vi "RoboticArm_Dashboard.vi"() -> ()   [LabVIEW 2019]
uses:
  <vilib>/MakerHub/Xbox-One-Controller/Public/Open by Index.vi
  <vilib>/vision/driver/NI_Vision_Acquisition_Software.lvlib
  <vilib>/MakerHub/Xbox-One-Controller/Private/Type Defs/Indicators/All Buttons Visual.ctl
  <vilib>/MakerHub/Xbox-One-Controller/Private/Type Defs/Indicators/A.ctl
  <vilib>/MakerHub/Xbox-One-Controller/Private/Type Defs/Indicators/B.ctl
  <vilib>/MakerHub/Xbox-One-Controller/Private/Type Defs/Indicators/X.ctl
  <vilib>/MakerHub/Xbox-One-Controller/Private/Type Defs/Indicators/Y.ctl
  <vilib>/MakerHub/Xbox-One-Controller/Private/Type Defs/Indicators/View.ctl
  <vilib>/MakerHub/Xbox-One-Controller/Private/Type Defs/Indicators/Menu.ctl
  <vilib>/MakerHub/Xbox-One-Controller/Private/Type Defs/Indicators/Thumbstick.ctl
  <vilib>/MakerHub/Xbox-One-Controller/Private/Type Defs/Indicators/Left Bumper.ctl
  <vilib>/MakerHub/Xbox-One-Controller/Private/Type Defs/Indicators/Right Bumper.ctl
  <vilib>/MakerHub/Xbox-One-Controller/Private/Type Defs/Indicators/All Axis Data.ctl
  <vilib>/MakerHub/Xbox-One-Controller/Private/Type Defs/Indicators/DPad Enum.ctl
  <vilib>/userDefined/High Color/IMAQdx.ctl
panel:
  in  "Session In":T1
  in  "Stop 2":bool
  out "Frame Rate":dbl(knob) scale=0.0..100.0
  out "Image":T2(plugin-control)
  out "Buffer Number":u32
  in  "Tab Control":T3(tab)
  in  "Blank Button":bool
  in  "PORT":dbl
  in  "IP-ADDRESS":string(combo)
  in  "Stop":bool
  in  "TCP/IP control":bool
  out "Servos Software Control":u8[](array[numeric])
  out "Manual?":bool
  in  "Servo control":bool
  out "Register values":i32[](array[numeric])
  in  "Servos manual angle":u8[](array[numeric])
  out "Value sent to Raspberry Pi":string
  out "hex integer string":string[](array[string])
  out "Raspberry pi feedback":string
  out "Stop?":bool
  out "Socket Error Out":errorcluster
  out "Gamepad Error Out":errorcluster
  out "Buttons":T4
  out "All Axis":T14
  in  "Device Index":i32
  in  "link B":dbl
  in  "link A":dbl
  out "Servo A":dbl(knob) scale=0.0..180.0
  in  "dist":dbl(knob) scale=50.0..250.0
  out "Servo B":dbl(knob) scale=0.0..180.0
  # "TCP/IP"
  # "Control Selector"
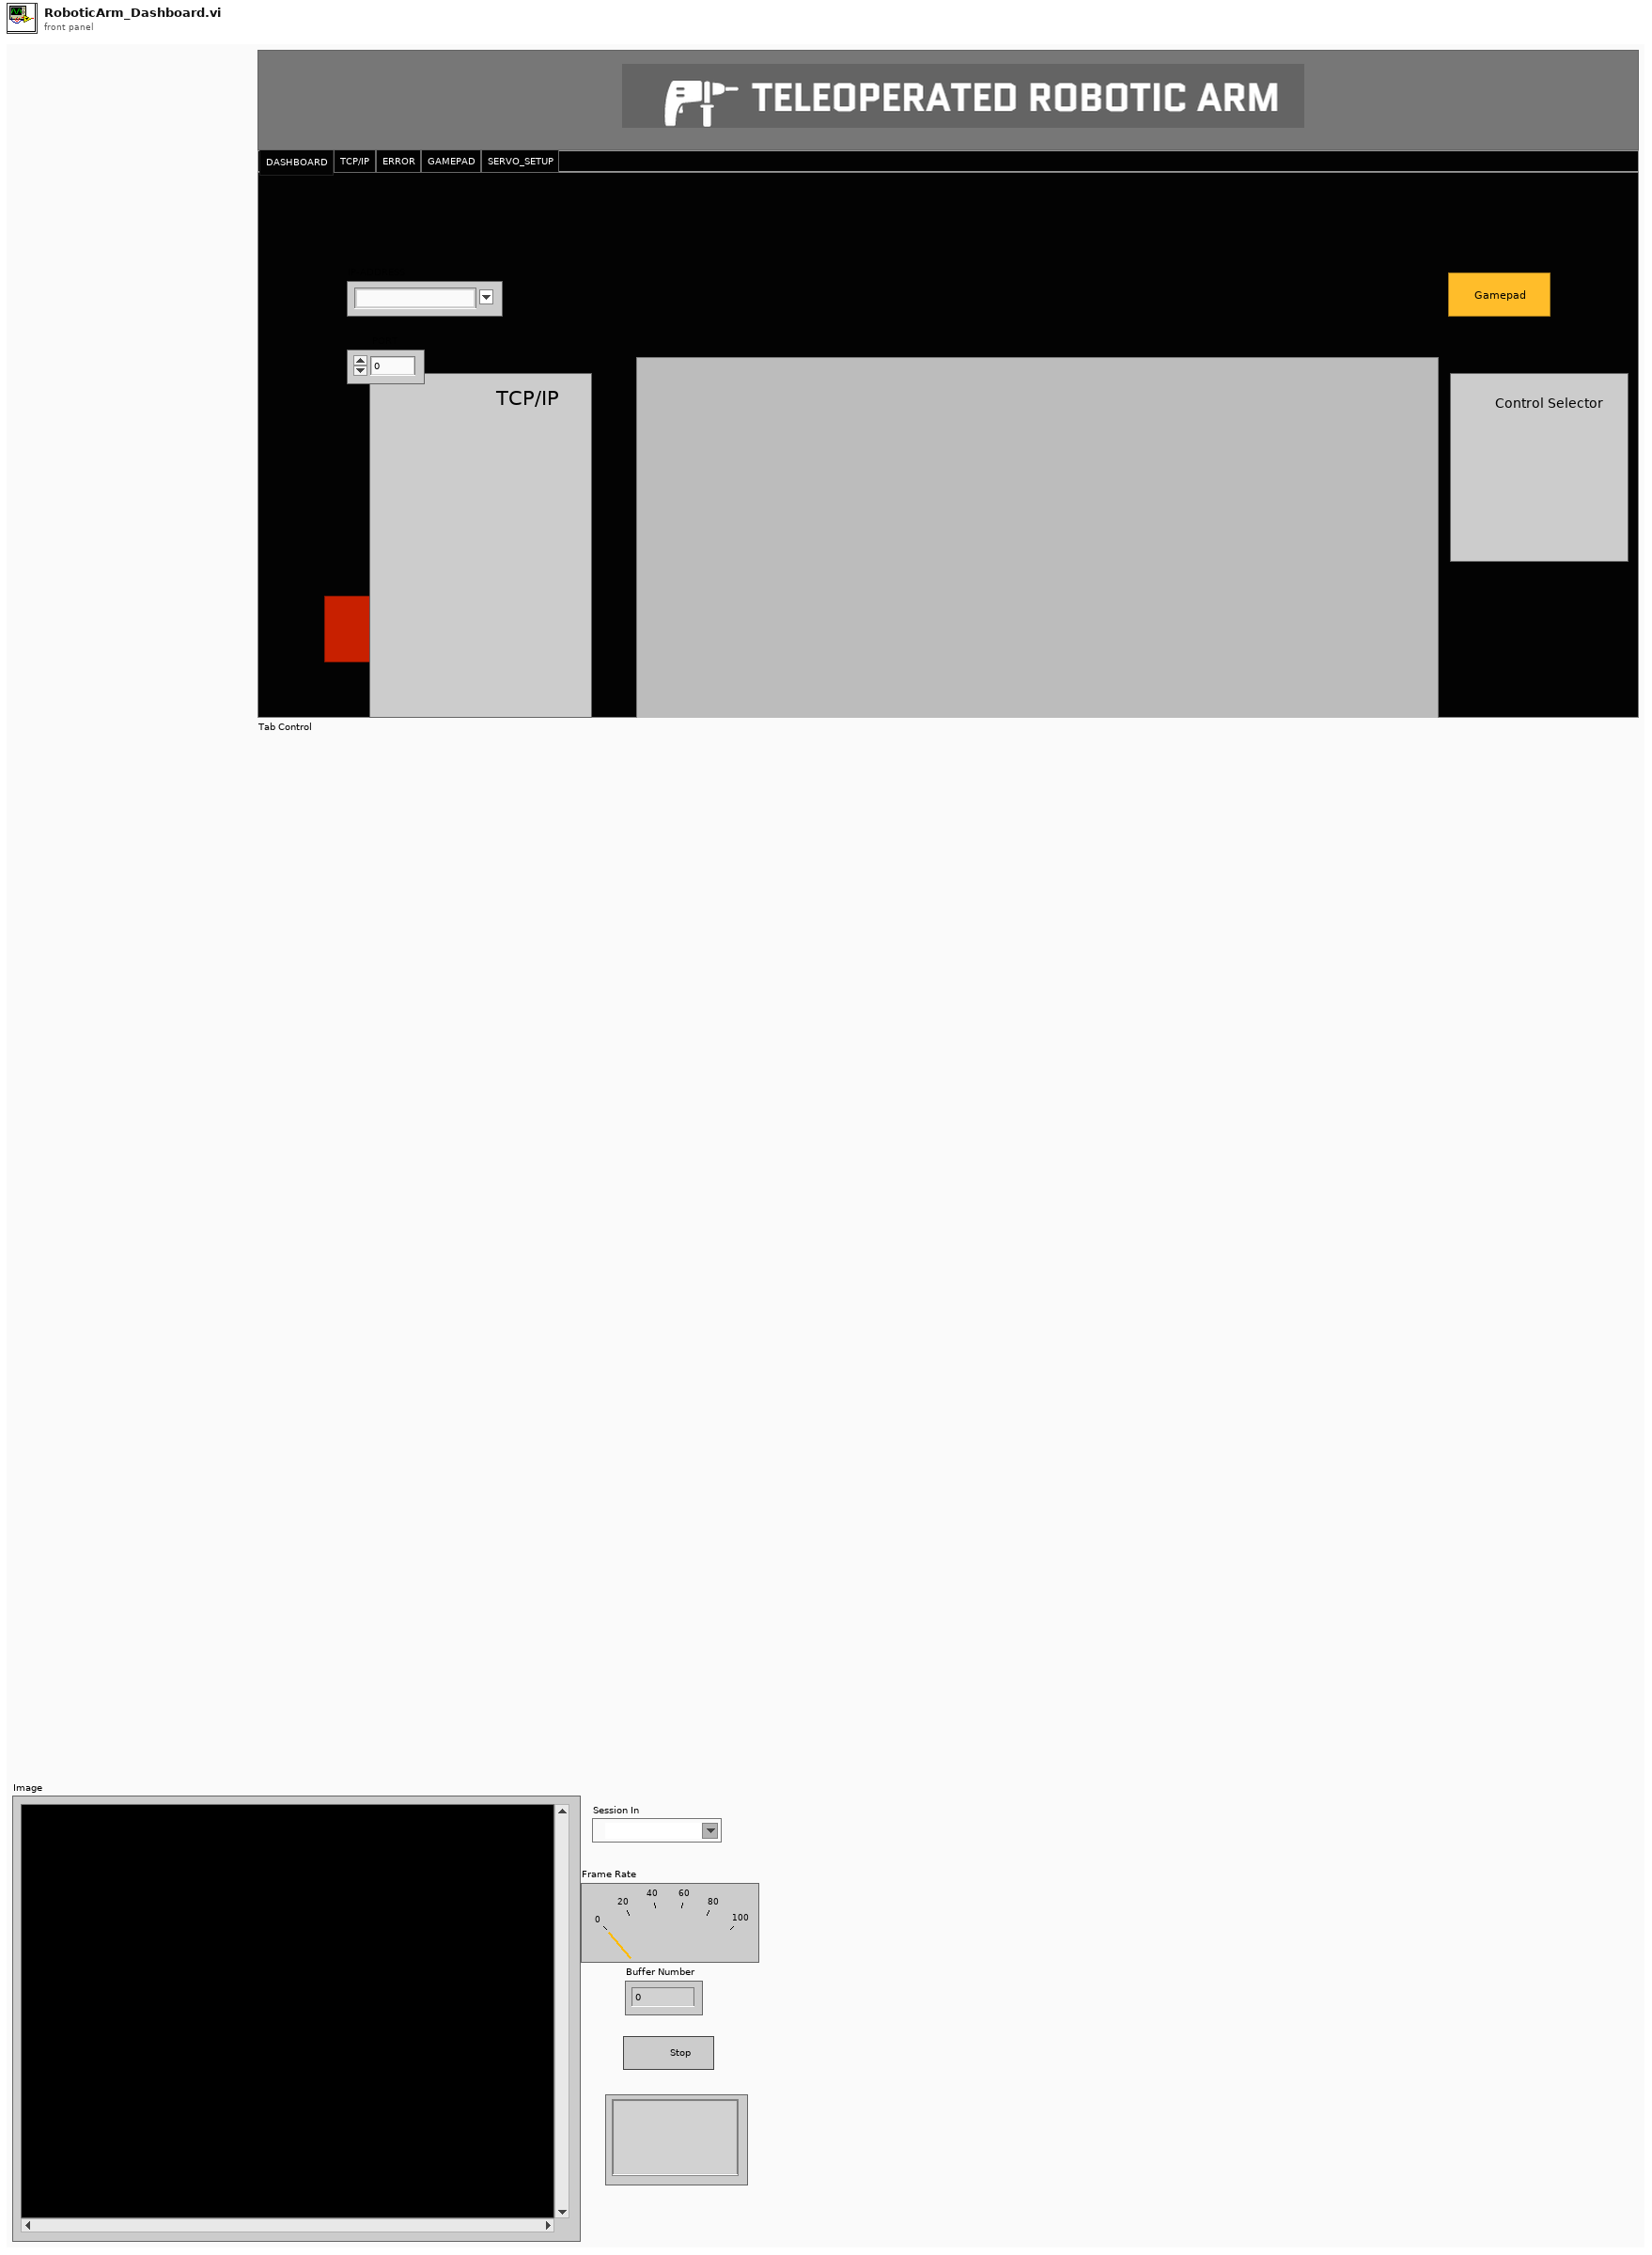
[diagram p1: front panel]
types:
  T1 = typedef "IMAQdx.ctl" = refnum<k21>
  T2 = typedef "IMAQ Image.ctl" = refnum<image>
  T3 = enum32{"DASHBOARD", "TCP/IP", "ERROR", "GAMEPAD", "SERVO_SETUP"}
  T4 = typedef "LMH-Xbox-One-Controller.lvlib/All Buttons Visual.ctl" = cluster{"A":T5, "B":T6, "X":T7, "Y":T8, "Left Bumper":T9, "Right Bumper":T10, "View Button":T11, "Menu Button":T12, "Left Stick":T13, "Right Stick":T13}
  T5 = typedef "LMH-Xbox-One-Controller.lvlib/A.ctl" = bool
  T6 = typedef "LMH-Xbox-One-Controller.lvlib/B.ctl" = bool
  T7 = typedef "LMH-Xbox-One-Controller.lvlib/X.ctl" = bool
  T8 = typedef "LMH-Xbox-One-Controller.lvlib/Y.ctl" = bool
  T9 = typedef "LMH-Xbox-One-Controller.lvlib/Left Bumper.ctl" = bool
  T10 = typedef "LMH-Xbox-One-Controller.lvlib/Right Bumper.ctl" = bool
  T11 = typedef "LMH-Xbox-One-Controller.lvlib/View.ctl" = bool
  T12 = typedef "LMH-Xbox-One-Controller.lvlib/Menu.ctl" = bool
  T13 = typedef "LMH-Xbox-One-Controller.lvlib/Thumbstick.ctl" = bool
  T14 = typedef "LMH-Xbox-One-Controller.lvlib/All Axis Data.ctl" = cluster{"Left Stick":cluster{"X Axis":i32, "Y Axis":i32}, "Right Stick":cluster{"X Axis":i32, "Y Axis":i32}, "Triggers":i32, "D-Pad":T15}
  T15 = typedef "LMH-Xbox-One-Controller.lvlib/DPad Enum.ctl" = enum16{"Idle", "Up", "Up / Right", "Right", "Down / Right", "Down", "Down / Left", "Left", "Up / Left"}
  T16 = typedef "LMH-Xbox-One-Controller.lvlib/Xbox One Controller Ref.ctl" = cluster{"Controller Ref":refnum<k1>, "Event Refnum":refnum<event-registration>, "Worker Ref":refnum<vi>}
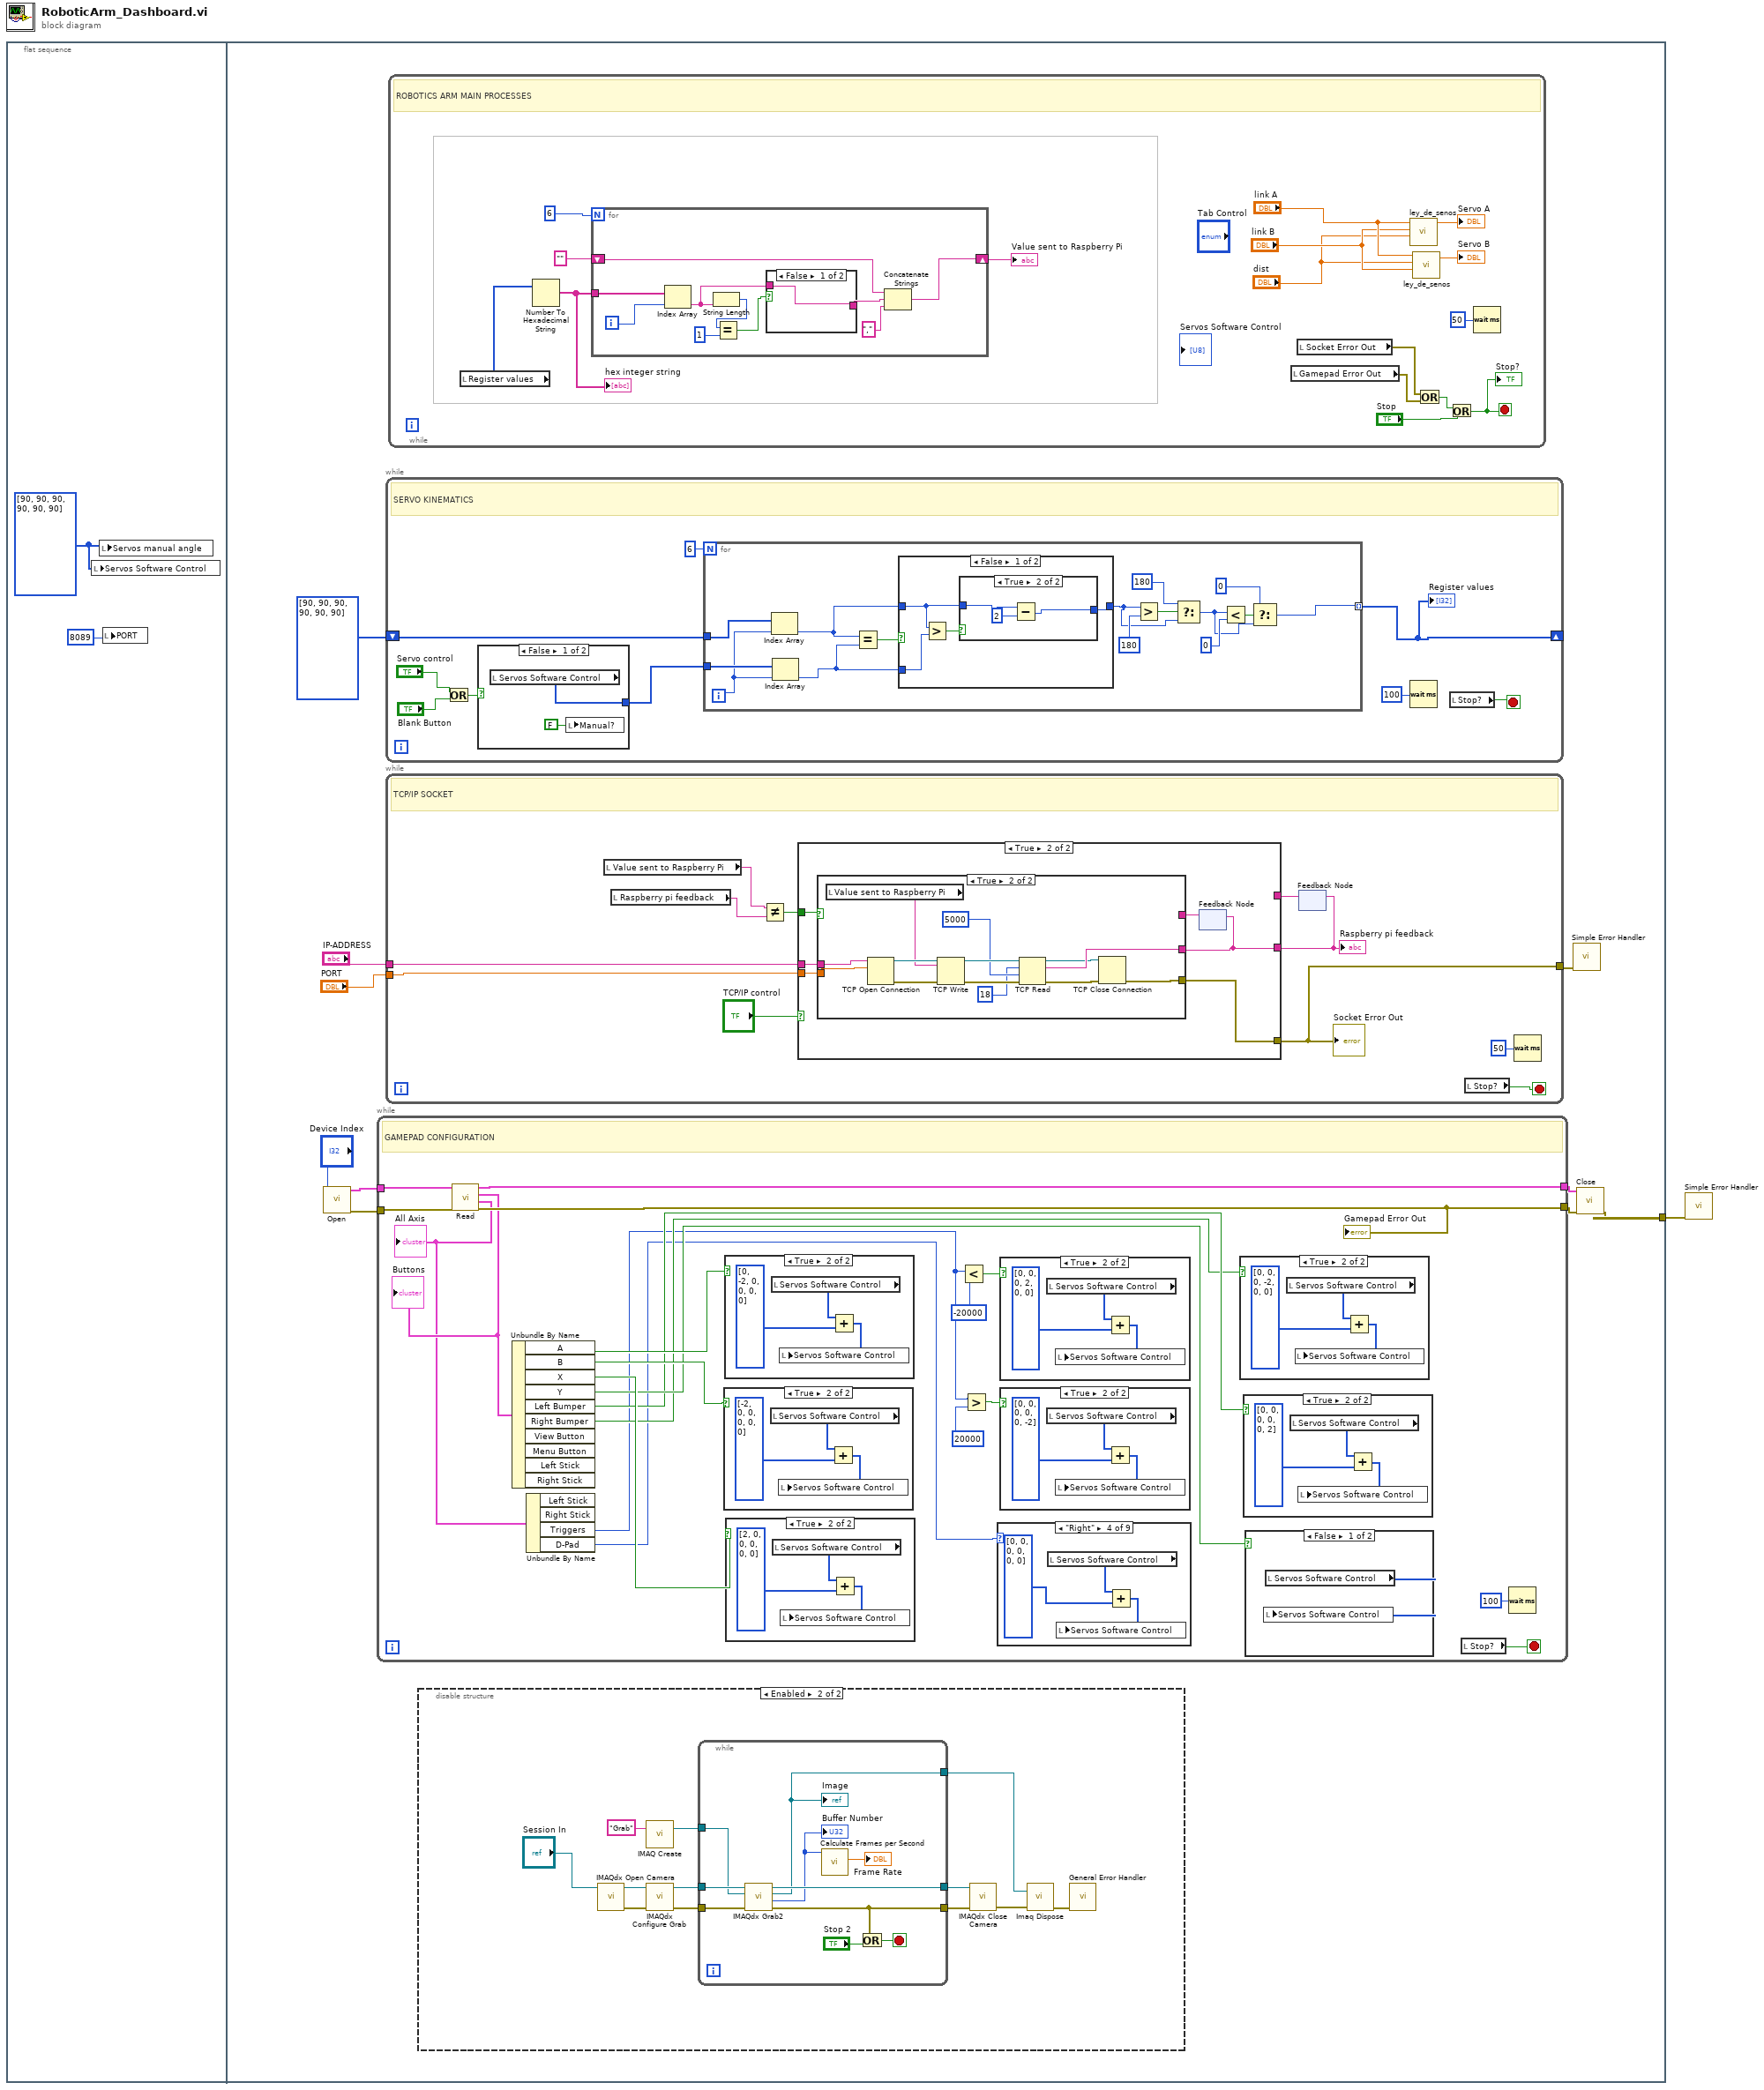
[diagram p0: block diagram]
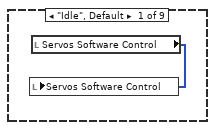
[diagram p3: hidden frame]
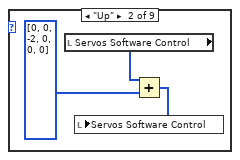
[diagram p4: hidden frame]
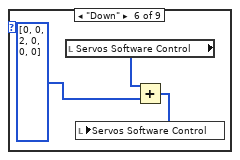
[diagram p7: hidden frame]
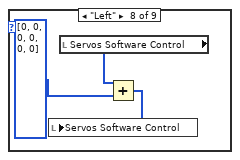
[diagram p9: hidden frame]
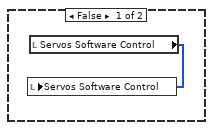
[diagram p11: hidden frame]
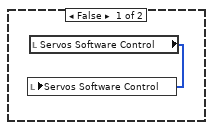
[diagram p12: hidden frame]
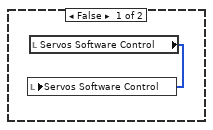
[diagram p13: hidden frame]
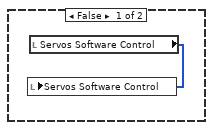
[diagram p14: hidden frame]
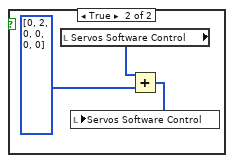
[diagram p15: hidden frame]
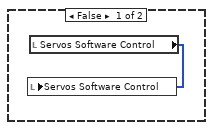
[diagram p16: hidden frame]
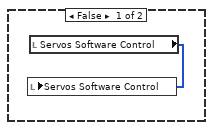
[diagram p17: hidden frame]
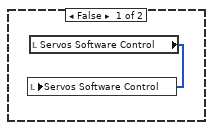
[diagram p18: hidden frame]
diagram:
  n1 = flat-sequence {
    tunnel: [w5] -> w1
    frame #0 {
      w2 = i32[] [90, 90, 90, 90, 90, 90]
      n2 = local write "Servos Software Control"(w2) -> ()
      n3 = local write "Servos manual angle"(w2) -> ()
      n4 = local write "PORT"(8089) -> ()
    }
    frame #1 {
      n5 = call-poly <vilib>:"Open.vi"("Device Index"="Device Index") -> ("Error Out"=w9:errorcluster, "Xbox One Controller Ref"=w10:T16)  [unwired: 8 in, 1 out]
      n6 = while {
        tunnel: w10 -> [w53]
        tunnel: w9 -> [w52]
        tunnel: [w50] -> w7
        tunnel: [w51] -> w6
        stop <- w55 stop-if-true
        # "GAMEPAD CONFIGURATION"
        n7 = call <vilib>:"Read.vi"("Error In"=w52, "Xbox One Controller Ref"=w53) -> ("Error Out"=w50:errorcluster, "All Axis"=w48:T14, "Buttons"=w49:T4, "Xbox One Controller Ref"=w51:T16)  [unwired: 6 in]
        "Gamepad Error Out" <- w50
        "Buttons" <- w49
        "All Axis" <- w48
        n8 = Unbundle By Name(w49) -> ("A"=w47:T5, "B"=w46:T6, "X"=w45:T7, "Y"=w44:T8, "Left Bumper"=w43:T9, "Right Bumper"=w42:T10)  [unwired: 4 out]
        n9 = Unbundle By Name(w48) -> ("Triggers"=w38:i32, "D-Pad"=w36:T15)  [unwired: 2 out]
        n10 = case shown="True" w46 {
          frame False {
            n11 = local read "Servos Software Control"() -> (w93:u8[])
            n12 = local write "Servos Software Control"(w93) -> ()
          }
          frame True {
            n13 = local read "Servos Software Control"() -> (w96:u8[])
            n14 = Add(x=w96, y=i32[] [-2, 0, 0, 0, 0, 0]) -> (x+y=w94:i32[])
            n15 = local write "Servos Software Control"(w94) -> ()
          }
        }
        n16 = case shown="True" w47 {
          frame False {
            n17 = local read "Servos Software Control"() -> (w97:u8[])
            n18 = local write "Servos Software Control"(w97) -> ()
          }
          frame True {
            n19 = local read "Servos Software Control"() -> (w100:u8[])
            n20 = Add(x=w100, y=i32[] [0, -2, 0, 0, 0, 0]) -> (x+y=w98:i32[])
            n21 = local write "Servos Software Control"(w98) -> ()
          }
        }
        n22 = case shown="True" w45 {
          frame False {
            n23 = local read "Servos Software Control"() -> (w89:u8[])
            n24 = local write "Servos Software Control"(w89) -> ()
          }
          frame True {
            n25 = local read "Servos Software Control"() -> (w92:u8[])
            n26 = Add(x=w92, y=i32[] [2, 0, 0, 0, 0, 0]) -> (x+y=w90:i32[])
            n27 = local write "Servos Software Control"(w90) -> ()
          }
        }
        n28 = Less?(x=w38, y=-20000) -> (x < y?=w39:bool)
        n29 = Greater?(x=w38, y=20000) -> (0:w41:bool)
        n30 = case shown="\"Right\"" w36 {
          frame "Idle", Default {
            n31 = local read "Servos Software Control"() -> (w56:u8[])
            n32 = local write "Servos Software Control"(w56) -> ()
          }
          frame "Up" {
            n33 = local read "Servos Software Control"() -> (w59:u8[])
            n34 = Add(x=w59, y=i32[] [0, 0, -2, 0, 0, 0]) -> (x+y=w57:i32[])
            n35 = local write "Servos Software Control"(w57) -> ()
          }
          frame "Up / Right" {
          }
          frame "Right" {
            n36 = local read "Servos Software Control"() -> (w61:u8[])
            n37 = Add(x=w61, y=i32[] [0, 0, 0, 0, 0, 0]) -> (x+y=w62:i32[])
            n38 = local write "Servos Software Control"(w62) -> ()
          }
          frame "Down / Right" {
          }
          frame "Down" {
            n39 = local read "Servos Software Control"() -> (w64:u8[])
            n40 = Add(x=w64, y=i32[] [0, 0, 2, 0, 0, 0]) -> (x+y=w65:i32[])
            n41 = local write "Servos Software Control"(w65) -> ()
          }
          frame "Down / Left" {
          }
          frame "Left" {
            n42 = local read "Servos Software Control"() -> (w67:u8[])
            n43 = Add(x=w67, y=i32[] [0, 0, 0, 0, 0, 0]) -> (x+y=w68:i32[])
            n44 = local write "Servos Software Control"(w68) -> ()
          }
          frame "Up / Left" {
          }
        }
        n45 = case shown="True" w39 {
          frame False {
            n46 = local read "Servos Software Control"() -> (w69:u8[])
            n47 = local write "Servos Software Control"(w69) -> ()
          }
          frame True {
            n48 = local read "Servos Software Control"() -> (w72:u8[])
            n49 = Add(x=w72, y=i32[] [0, 0, 0, 2, 0, 0]) -> (x+y=w70:i32[])
            n50 = local write "Servos Software Control"(w70) -> ()
          }
        }
        n51 = case shown="True" w41 {
          frame False {
            n52 = local read "Servos Software Control"() -> (w73:u8[])
            n53 = local write "Servos Software Control"(w73) -> ()
          }
          frame True {
            n54 = local read "Servos Software Control"() -> (w76:u8[])
            n55 = Add(x=w76, y=i32[] [0, 0, 0, 0, 0, -2]) -> (x+y=w74:i32[])
            n56 = local write "Servos Software Control"(w74) -> ()
          }
        }
        n57 = case shown="True" w42 {
          frame False {
            n58 = local read "Servos Software Control"() -> (w77:u8[])
            n59 = local write "Servos Software Control"(w77) -> ()
          }
          frame True {
            n60 = local read "Servos Software Control"() -> (w80:u8[])
            n61 = Add(x=w80, y=i32[] [0, 0, 0, -2, 0, 0]) -> (x+y=w78:i32[])
            n62 = local write "Servos Software Control"(w78) -> ()
          }
        }
        n63 = case shown="True" w43 {
          frame False {
            n64 = local read "Servos Software Control"() -> (w81:u8[])
            n65 = local write "Servos Software Control"(w81) -> ()
          }
          frame True {
            n66 = local read "Servos Software Control"() -> (w84:u8[])
            n67 = Add(x=w84, y=i32[] [0, 0, 0, 0, 0, 2]) -> (x+y=w82:i32[])
            n68 = local write "Servos Software Control"(w82) -> ()
          }
        }
        n69 = case shown="False" w44 {
          frame False {
            n70 = local read "Servos Software Control"() -> (w85:u8[])
            n71 = local write "Servos Software Control"(w85) -> ()
          }
          frame True {
            n72 = local read "Servos Software Control"() -> (w88:u8[])
            n73 = Add(x=w88, y=i32[] [0, 2, 0, 0, 0, 0]) -> (x+y=w86:i32[])
            n74 = local write "Servos Software Control"(w86) -> ()
          }
        }
        n75 = local read "Stop?"() -> (w55:bool)
        n76 = Wait (ms)(milliseconds to wait=u32 100) -> ()  [unwired: 1 out]
      }
      n77 = while {
        shift-right: [w133] -> _
        shift-left: i32[] [90, 90, 90, 90, 90, 90] -> [w137]
        stop <- w138 stop-if-true
        # "SERVO KINEMATICS"
        n78 = Or(x="Servo control", y="Blank Button") -> (x .or. y?=w136:bool)
        n79 = case shown="False" w136 {
          tunnel: [w143 "Servos manual angle"] -> w140
          frame False {
            n80 = local read "Servos Software Control"() -> (w143:u8[])
            n81 = local write "Manual?"(FALSE ("Manual?")) -> ()
          }
          frame True {
            "Manual?" <- TRUE ("Manual?")
          }
        }
        n82 = for {
          N: 6 -> [_]
          tunnel: w137 -> [w159]
          tunnel: w140 -> [w157]
          tunnel: [w146] -> w133 mode=indexing
          i -> [w156]
          n83 = Index Array(array=w159, index=w156) -> (element=w158:i32)
          n84 = Index Array(array=w157, index=w156) -> (element=w155:u8)
          n85 = Equal?(x=w158, y=w155) -> (x = y?=w160:bool)
          n86 = case shown="False" w160 {
            tunnel: w158 -> [w162 w171]
            tunnel: [w161 w171] -> w151
            tunnel: w155 -> [w163 _]
            frame False {
              n87 = Greater?(x=w162, y=w163) -> (0:w164:bool)
              n88 = case shown="True" w164 {
                tunnel: w162 -> [w166 w169]
                tunnel: [w167 w170] -> w161
                frame False {
                  n89 = Add(x=w166, y=2) -> (x+y=w167:i32)
                }
                frame True {
                  n90 = Subtract(x=w169, y=2) -> (x-y=w170:i32)
                }
              }
            }
            frame True {
            }
          }
          n91 = Greater?(x=w151, y=180) -> (0:w153:bool)
          n92 = Select(t=u8 180, s=w153, f=w151) -> (s? t:f=w147:i32)
          n93 = Less?(x=w147, y=0) -> (x < y?=w149:bool)
          n94 = Select(t=u8 0, s=w149, f=w147) -> (s? t:f=w146:i32)
        }
        "Register values" <- w133
        n95 = Wait (ms)(milliseconds to wait=u32 100) -> ()  [unwired: 1 out]
        n96 = local read "Stop?"() -> (w138:bool)
      }
      n97 = while {
        tunnel: "IP-ADDRESS" -> [w109]
        tunnel: "PORT" -> [w108]
        tunnel: [w104] -> w8
        stop <- w111 stop-if-true
        # "TCP/IP SOCKET"
        n98 = local read "Value sent to Raspberry Pi"() -> (w102:string)
        n99 = local read "Raspberry pi feedback"() -> (w101:string)
        n100 = Not Equal?(x=w102, y=w101) -> (x != y?=w103:bool)
        n101 = feedback #1() -> (w105:string)  [unwired: 1 in]
        n102 = case shown="True" "TCP/IP control" {
          tunnel: w109 -> [_ w118]
          tunnel: w108 -> [_ w117]
          tunnel: [w112 w115] -> w106
          tunnel: [_ w114] -> w104
          tunnel: w105 -> [w112 _]
          tunnel: w103 -> [_ w113]
          frame False {
          }
          frame True {
            n103 = feedback #2() -> (w116:string)  [unwired: 1 in]
            n104 = case shown="True" w113 {
              tunnel: [w119 w132] -> w115
              tunnel: [_ w131] -> w114
              tunnel: w118 -> [_ w122]
              tunnel: w117 -> [_ w121]
              tunnel: w116 -> [w119 _]
              frame False {
              }
              frame True {
                n105 = local read "Value sent to Raspberry Pi"() -> (w120:string)
                n106 = TCP Open Connection(address=w122, remote port or service name=w121) -> (connection ID=w127:refnum<k5>, error out=w128:errorcluster)  [unwired: 3 in]
                n107 = TCP Write(connection ID=w127, data in=w120, error in (no error)=w128) -> (connection ID out=w125:refnum<k5>, error out=w126:errorcluster)  [unwired: 1 in, 1 out]
                n108 = TCP Read(connection ID=w125, bytes to read=18, error in (no error)=w126, 9:5000 ("timeout ms (25000)")) -> (connection ID out=w129:refnum<k5>, data out=w132:string, error out=w130:errorcluster)  [unwired: 1 in]
                n109 = TCP Close Connection(connection ID=w129, error in (no error)=w130) -> (error out=w131:errorcluster)  [unwired: 1 in, 1 out]
              }
            }
            n110 = feedback-in #2(w115) -> ()
          }
        }
        "Raspberry pi feedback" <- w106
        "Socket Error Out" <- w104
        n111 = feedback-in #1(w106) -> ()
        n112 = local read "Stop?"() -> (w111:bool)
        n113 = Wait (ms)(milliseconds to wait=u32 50) -> ()  [unwired: 1 out]
      }
      n114 = while {
        stop <- w177 stop-if-true
        # "ROBOTICS ARM MAIN PROCESSES"
        n115 = local read "Register values"() -> (w179:i32[])
        n116 = Number To Hexadecimal String(2:w179) -> (0:w180:string[])  [unwired: 1 in]
        "hex integer string" <- w180
        n117 = for {
          N: 6 -> [_]
          shift-right: [w194] -> w178
          shift-left: "" -> [w195]
          tunnel: w180 -> [w189]
          i -> [w197]
          n118 = Index Array(array=w189, index=w197) -> (element=w188:string)
          n119 = String Length(string=w188) -> (length=w193:i32)
          n120 = Equal?(x=w193, y=1) -> (x = y?=w192:bool)
          n121 = case shown="False" w192 {
            tunnel: [w198 w200] -> w190
            tunnel: w188 -> [w198 w199]
            frame False {
            }
            frame True {
              n122 = Concatenate Strings("0" ("string"), w199) -> (w200:string)
            }
          }
          n123 = Concatenate Strings(w195, w190, "," ("string")) -> (w194:string)
        }
        "Value sent to Raspberry Pi" <- w178
        n124 = local read "Gamepad Error Out"() -> (w173:errorcluster)
        n125 = local read "Socket Error Out"() -> (w174:errorcluster)
        n126 = call "ley_de_senos.vi"("ady2"="dist", "opuesto"="link B", "ady1"="link A") -> ("angulo"=→"Servo A":dbl)  [unwired: 8 in]
        n127 = call "ley_de_senos.vi"("ady2"="link B", "opuesto"="dist", "ady1"="link A") -> ("angulo"=→"Servo B":dbl)  [unwired: 8 in]
        n128 = Or(x=w174, y=w173) -> (x .or. y?=w175:bool)
        n129 = Or(x=w175, y="Stop") -> (x .or. y?=w177:bool)
        "Stop?" <- w177
        n130 = Wait (ms)(milliseconds to wait=u32 50) -> ()  [unwired: 1 out]
      }
      n131 = disable-structure shown="Enabled" {
        frame Disabled {
        }
        frame Enabled {
          n132 = call <vilib>:"IMAQdx Open Camera.vi"("Session In"="Session In") -> ("error out"=w20:errorcluster, "Session Out"=w19:T1)  [unwired: 2 in, 7 out]
          n133 = call "IMAQ Create"("Image Name"="Grab") -> ("New Image"=w25:T2)  [unwired: 3 in, 2 out]
          n134 = call <vilib>:"IMAQdx Configure Grab.vi"("error in"=w20, "Session In"=w19) -> ("error out"=w23:errorcluster, "Session Out"=w24:T1)  [unwired: 1 in, 7 out]
          n135 = while {
            tunnel: [w30] -> w22
            tunnel: w23 -> [w32]
            tunnel: w24 -> [w33]
            tunnel: [w27] -> w21
            tunnel: w25 -> [w31]
            tunnel: [w26] -> w18
            stop <- w35 stop-if-true
            n136 = call <vilib>:"IMAQdx Grab2.vi"("error in"=w32, "Image In"=w31, "Session In"=w33) -> ("error out"=w27:errorcluster, "Buffer Number Out"=w28:u32, "Image Out"=w26:T2, "Session Out"=w30:T1)  [unwired: 5 in]
            "Image" <- w26
            "Buffer Number" <- w28
            n137 = call <vilib>:"Calculate Frames per Second.vi"("Buffer Number"=w28) -> ("Processed Frames/s"=→"Frame Rate":dbl)  [unwired: 8 in, 2 out]
            n138 = Or(x=w27, y="Stop 2") -> (x .or. y?=w35:bool)
          }
          n139 = call <vilib>:"IMAQdx Close Camera.vi"("error in"=w21, "Session In"=w22) -> ("error out"=w17:errorcluster)  [unwired: 9 out]
          n140 = call "Imaq Dispose"("Image"=w18, "error in (no error)"=w17) -> ("error out"=w16:errorcluster)  [unwired: 4 in]
          n141 = call <vilib>:"General Error Handler.vi"("error in (no error)"=w16) -> ()  [unwired: 2 in, 13 out]
        }
      }
      n142 = call <vilib>:"Simple Error Handler.vi"("error in (no error)"=w8) -> ()  [unwired: 4 in, 5 out]
      n143 = call <vilib>:"Close.vi"("Error In"=w7, "Xbox One Controller Ref"=w6) -> ("Error Out"=w5:errorcluster)  [unwired: 9 in]
    }
  }
  n144 = call <vilib>:"Simple Error Handler.vi"("error in (no error)"=w1) -> ()  [unwired: 4 in, 5 out]
